vi "Log File.vi"(10 "new file path (Not A Path if cancelled)":path, 11 "Active Input":T1=enum."None") -> ()   [LabVIEW 2024]
uses:
  Active Input.ctl
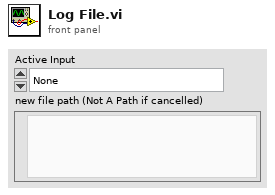
[diagram p1: front panel]
types:
  T1 = typedef "Active Input.ctl" = enum16{"Alarm, Bypass & Tamper", "Bypass & Tamper", "Alarm & Tamper", "Alarm & Bypass", "Tamper", "Bypass", "Alarm", "None"}
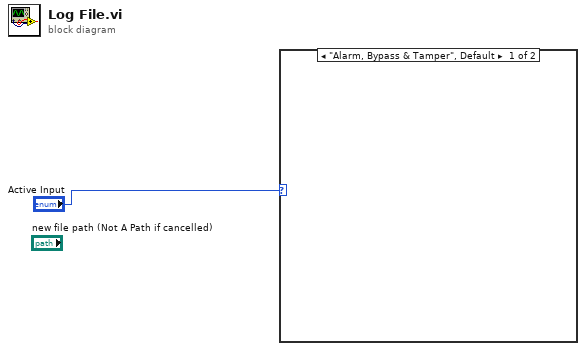
[diagram p0: block diagram]
diagram:
  n1 = case shown="\"Alarm, Bypass & Tamper\", Default" "Active Input" {
    frame "Alarm, Bypass & Tamper", Default {
    }
    frame "Bypass & Tamper" {
    }
  }
